vi "LEDColorNumberToColor.vi"(11 "ColorNumber":dbl) -> (3 "Color":u32(colorbox))   [LabVIEW 2018]
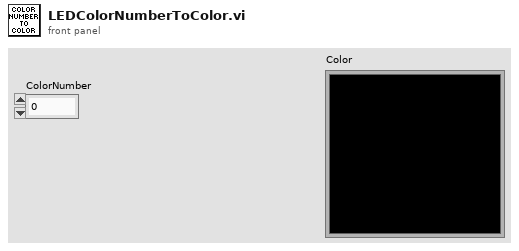
[diagram p1: front panel]
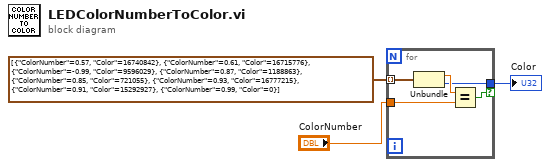
[diagram p0: block diagram]
diagram:
  n1 = for {
    tunnel: "ColorNumber" -> [w7]
    tunnel: cluster{"ColorNumber":dbl, "Color":u32}[] [{"ColorNumber"=0.57, "Color"=16740842}, {"ColorNumber"=0.61, "Color"=16715776}, {"ColorNumber"=-0.99, "Color"=9596029}, {"ColorNumber"=0.87, "Color"=1188863}, {"ColorNumber"=0.85, "Color"=721055}, {"ColorNumber"=0.93, "Color"=16777215}, {"ColorNumber"=0.91, "Color"=15292927}, {"ColorNumber"=0.99, "Color"=0}] -> [w8] mode=indexing
    tunnel: [w5] -> w1 if=w4
    n2 = Unbundle(w8) -> ("ColorNumber"=w6:dbl, "Color"=w5:u32)
    n3 = Equal?(x=w6, y=w7) -> (x = y?=w4:bool)
  }
  "Color" <- w1
